vi "字串轉換.vi"(2 "error in (no error)":errorcluster, 3 "字串(I)":string) -> (0 "error out":errorcluster, 1 "字串(O)":string)   [LabVIEW 2015]
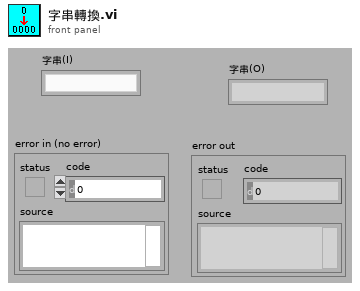
[diagram p1: front panel]
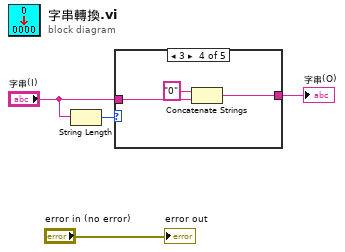
[diagram p0: block diagram]
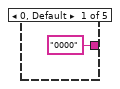
[diagram p2: hidden frame]
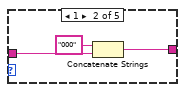
[diagram p3: hidden frame]
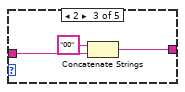
[diagram p4: hidden frame]
diagram:
  n1 = String Length(string="字串(I)") -> (length=w4:i32)
  n2 = case shown="3" w4 {
    tunnel: "字串(I)" -> [_ w8 w10 w13 w15]
    tunnel: ["0000" ("字串(I)") w6 w11 w14 w15] -> w2
    frame 0, Default {
    }
    frame 1 {
      n3 = Concatenate Strings("000", w8) -> (w6:string)
    }
    frame 2 {
      n4 = Concatenate Strings("00", w10) -> (w11:string)
    }
    frame 3 {
      n5 = Concatenate Strings("0", w13) -> (w14:string)
    }
    frame 4 {
    }
  }
  "字串(O)" <- w2
  "error out" <- "error in (no error)"
